vi "Handle Exception.vi"(7 "Processing In":refnum<class "Processing.lvclass">, 8 "error in (no error)":errorcluster, 11 "NoControllerException in":refnum<class "NoControllerException.lvclass">) -> (0 "error out":errorcluster, 5 "Processing":refnum<class "Processing.lvclass">)   [LabVIEW 2020, in "HTTP Server.lvlib" / "NoControllerException.lvclass"]
uses:
  NoControllerException.lvclass
  Processing/Processing.lvclass
  NoControllerException.lvclass/NoControllerException.ctl
  <vilib>/Utility/error.llb/DialogType.ctl
  Processing/Processing.lvclass/Processing.ctl
  lv-http-util/HTTP Utils/Response/Response.lvclass
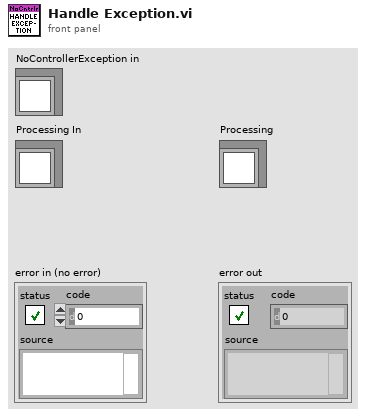
[diagram p1: front panel]
types:
  T1 = typedef "DialogType.ctl" = u16
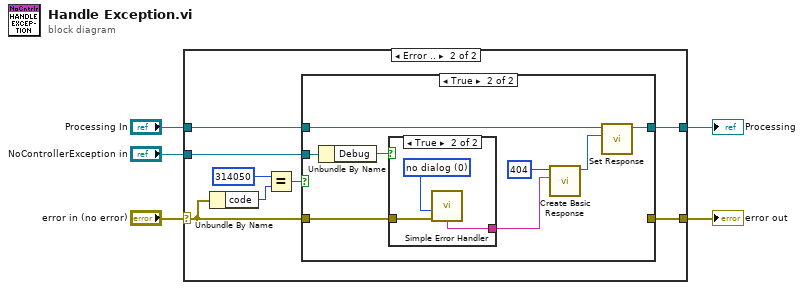
[diagram p0: block diagram]
diagram:
  n1 = case shown="Error .." "error in (no error)" {
    selector: "error in (no error)" -> [w7 w13]
    tunnel: [w7 w11] -> w4
    tunnel: [w6 w10] -> w3
    tunnel: "NoControllerException in" -> [_ w9]
    tunnel: "Processing In" -> [w6 w8]
    frame No Error {
    }
    frame Error {
      n2 = Unbundle By Name(w13) -> ("code"=w15:i32)
      n3 = Equal?(x=314050, y=w15) -> (x = y?=w12:bool)
      n4 = case shown="True" w12 {
        tunnel: w13 -> [w17 w22]
        tunnel: [w17 _] -> w11
        tunnel: [w16 w18] -> w10
        tunnel: w9 -> [_ w24]
        tunnel: w8 -> [w16 w20]
        frame False {
        }
        frame True {
          n5 = Unbundle By Name(w24) -> ("Debug"=w23:bool)
          n6 = case shown="True" w23 {
            tunnel: w22 -> [_ w27]
            tunnel: [_ w26] -> w21
            frame False {
            }
            frame True {
              w28 = T1 0 items=["no dialog", "OK message", "continue or stop message", "OK message + warnings", "continue/stop + warnings"] ("type of dialog (OK msg:1)")
              n7 = call <vilib>:"Simple Error Handler.vi"("type of dialog (OK msg:1)"=w28, "error in (no error)"=w27) -> ("message"=w26:string)  [unwired: 3 in, 4 out]
            }
          }
          n8 = call "Create Basic Response.vi"("Payload"=w21, "Status Code"=u16 404) -> ("Response out"=w19:refnum<class "Response.lvclass">)  [unwired: 8 in, 1 out]
          n9 = call "Set Response.vi"("Response"=w19, "Processing in"=w20) -> ("Processing out"=w18:refnum<class "Processing.lvclass">)  [unwired: 9 in]
        }
      }
    }
  }
  "error out" <- w4
  "Processing" <- w3
